vi "Read OOB TX.vi"(8 "error in (no error)":errorcluster, 11 "CIFTemplatePlugin in":refnum<class "TemplatePlugin.lvclass">) -> (0 "error out":errorcluster, 3 "CIFTemplatePlugin out":refnum<class "TemplatePlugin.lvclass">)   [LabVIEW 2021, in "TemplatePlugin.lvclass"]
uses:
  TemplatePlugin.lvclass
  TemplatePlugin.lvclass/TemplatePlugin.ctl
  OOB/OOB_Tx/TemplateOOB_Tx.lvclass
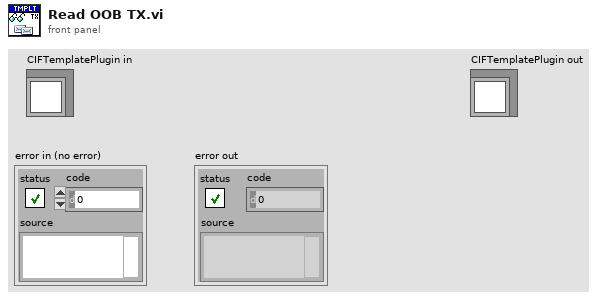
[diagram p1: front panel]
types:
  T1 = typedef "TemplateOOB_Tx.lvclass/OOB Commands.ctl" = enum8{"Update Data"}
  T2 = typedef "TemplateOOB_Tx.lvclass/Cyclic Data.ctl" = cluster{"Result":i32}
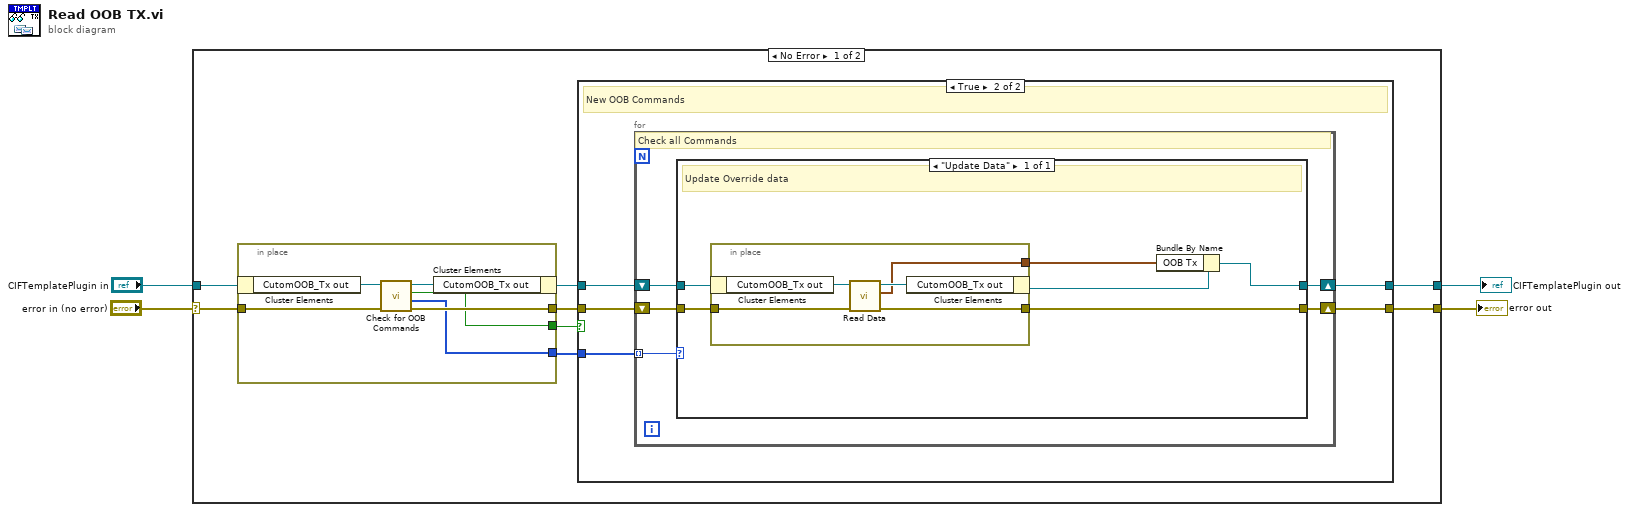
[diagram p0: block diagram]
diagram:
  n1 = case shown="No Error" "error in (no error)" {
    selector: "error in (no error)" -> [w11 w43]
    tunnel: [w5 w43] -> w3
    tunnel: [w7 w42] -> w1
    tunnel: "CIFTemplatePlugin in" -> [w12 w42]
    frame No Error {
      n2 = in-place {
        in-place-border: w11 -> [w40]
        in-place-border: [w38] -> w6
        in-place-border: [w37] -> w9
        in-place-border: [w36] -> w10
        n3 = in-place-cluster #1(w12) -> ("CutomOOB_Tx out"=w41:refnum<class "TemplateOOB_Tx.lvclass">)
        n4 = call "Check for OOB Commands.vi"("error in (no error)"=w40, "CutomOOB_Tx in"=w41) -> ("error out"=w38:errorcluster, "Commands"=w37:T1[], "New Commands"=w36:bool, "CutomOOB_Tx out"=w39:refnum<class "TemplateOOB_Tx.lvclass">)  [unwired: 6 in]
        n5 = in-place-cluster #1("CutomOOB_Tx out"=w39) -> (w8:refnum<class "TemplatePlugin.lvclass">)
      }
      n6 = case shown="True" w10 {
        tunnel: w9 -> [_ w19]
        tunnel: w8 -> [w14 w18]
        tunnel: [w14 w16] -> w7
        tunnel: w6 -> [w13 w17]
        tunnel: [w13 w15] -> w5
        frame False {
          # "No new OOB Commands"
        }
        frame True {
          # "New OOB Commands"
          n7 = for {
            tunnel: w19 -> [w24] mode=indexing
            shift-right: [w21] -> w16
            shift-left: w18 -> [w22]
            shift-right: [w20] -> w15
            shift-left: w17 -> [w23]
            # "Check all Commands"
            n8 = case shown="\"Update Data\"" w24 {
              tunnel: w23 -> [w29]
              tunnel: w22 -> [w30]
              tunnel: [w26] -> w21
              tunnel: [w28] -> w20
              frame "Update Data" {
                # "Update Override data"
                n9 = in-place {
                  in-place-border: w29 -> [w34]
                  in-place-border: [w32] -> w28
                  in-place-border: [w31] -> w25
                  n10 = in-place-cluster #2(w30) -> ("CutomOOB_Tx out"=w35:refnum<class "TemplateOOB_Tx.lvclass">)
                  n11 = call "Read Data.vi"("error in"=w34, "CutomOOB_Tx in"=w35) -> ("error out"=w32:errorcluster, "Data"=w31:T2, "CutomOOB_Tx out"=w33:refnum<class "TemplateOOB_Tx.lvclass">)  [unwired: 7 in]
                  n12 = in-place-cluster #2("CutomOOB_Tx out"=w33) -> (w27:refnum<class "TemplatePlugin.lvclass">)
                }
                n13 = Bundle By Name(cluster=w27, "OOB Tx"=w25) -> (w26:refnum<class "TemplatePlugin.lvclass">)
              }
            }
          }
        }
      }
    }
    frame Error {
    }
  }
  "error out" <- w3
  "CIFTemplatePlugin out" <- w1
